vi "MyAnd.vi"(10 "B":bool, 11 "A":bool) -> (3 "A and B":bool)   [LabVIEW 2020]
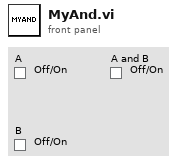
[diagram p1: front panel]
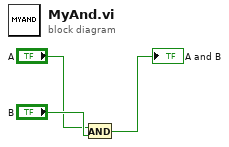
[diagram p0: block diagram]
diagram:
  n1 = And(x="A", y="B") -> (x .and. y?=→"A and B":bool)
